vi "Configure Bias.vi"(7 "DC Bias State (F:Disable)":bool, 8 "error in (no error)":errorcluster, 9 "DC Bias Type (0: Voltage)":u16(ring) items=["Voltage", "Current"], 10 "DC Bias Level (0.0 V)":dbl, 11 "Agilent 428x in":refnum<class "Agilent 428x.lvclass">) -> (0 "error out":errorcluster, 3 "Agilent 428x out":refnum<class "Agilent 428x.lvclass">)   [LabVIEW 2020, in "Agilent 428x.lvclass"]
uses:
  Agilent 428x.lvclass
  C:/Sandbox/RF Bench/Source Code/WiSpry Test Framework/Instruments/Instrument.lvclass
  Instrument.lvclass/Instrument.ctl
  Instrument.lvclass
  <instrlib>/Agilent 428X Series/Agilent 428X Series.lvlib
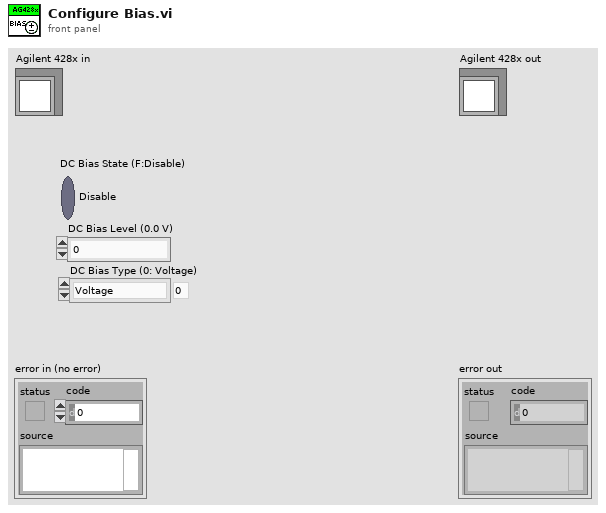
[diagram p1: front panel]
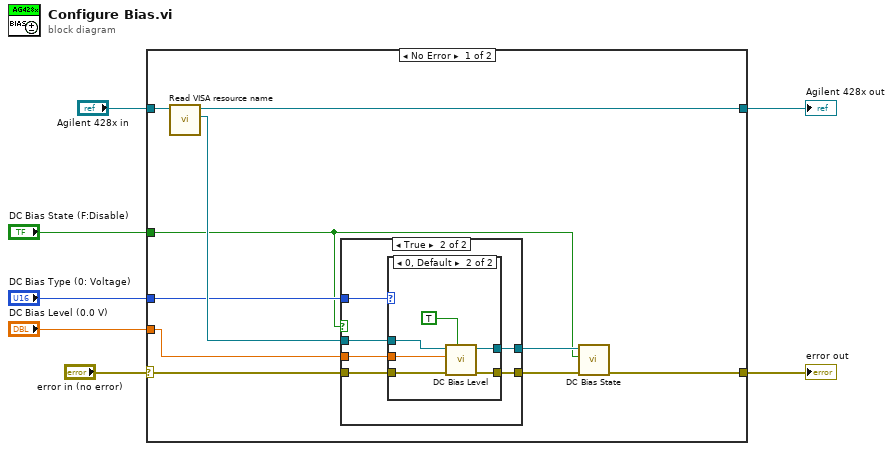
[diagram p0: block diagram]
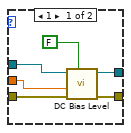
[diagram p3: hidden frame]
diagram:
  n1 = case shown="No Error" "error in (no error)" {
    selector: "error in (no error)" -> [w13 w39]
    tunnel: [w10 w39] -> w6
    tunnel: [w16 w38] -> w5
    tunnel: "Agilent 428x in" -> [w17 w38]
    tunnel: "DC Bias Level (0.0 V)" -> [w14 _]
    tunnel: "DC Bias State (F:Disable)" -> [w8 _]
    tunnel: "DC Bias Type (0: Voltage)" -> [w9 _]
    frame No Error {
      n2 = call "Read VISA resource name.vi"("Instrument in"=w17) -> ("VISA resource name"=w15:refnum<visa-resource-name>, "Instrument out"=w16:refnum<class "Agilent 428x.lvclass">)  [unwired: 9 in]
      n3 = case shown="True" w8 {
        tunnel: w15 -> [w18 w25]
        tunnel: w14 -> [_ w24]
        tunnel: w13 -> [w19 w23]
        tunnel: [w18 w22] -> w12
        tunnel: [w19 w21] -> w11
        tunnel: w9 -> [_ w20]
        frame False {
        }
        frame True {
          n4 = case shown="0, Default" w20 {
            tunnel: w25 -> [w31 w37]
            tunnel: w24 -> [w26 w36]
            tunnel: w23 -> [w30 w35]
            tunnel: [w28 w33] -> w22
            tunnel: [w27 w32] -> w21
            frame 1 {
              n5 = call <instrlib>:"DC Bias Level.vi"("Level Selector (T: Volt)"=FALSE, "error in (no error)"=w30, "Current Level (A) (0.0)"=w26, "VISA resource name"=w31) -> ("error out"=w27:errorcluster, "VISA resource name out"=w28:refnum<visa-resource-name>)  [unwired: 6 in]
            }
            frame 0, Default {
              n6 = call <instrlib>:"DC Bias Level.vi"("Level Selector (T: Volt)"=TRUE, "error in (no error)"=w35, "Voltage Level (V) (0.0)"=w36, "VISA resource name"=w37) -> ("error out"=w32:errorcluster, "VISA resource name out"=w33:refnum<visa-resource-name>)  [unwired: 6 in]
            }
          }
        }
      }
      n7 = call <instrlib>:"DC Bias State.vi"("error in (no error)"=w11, "State (F: Off)"=w8, "VISA resource name"=w12) -> ("error out"=w10:errorcluster)  [unwired: 7 in, 1 out]
    }
    frame Error {
    }
  }
  "error out" <- w6
  "Agilent 428x out" <- w5
